vi "Get Cursor X positions.vi"(8 "error in":errorcluster, 11 "XY Graph Ref":refnum<vi>) -> (0 "error out":errorcluster, 1 "Cursors":cluster{"Left":dbl, "Right":dbl, "Span":dbl}, 2 "Right":dbl, 3 "Left":dbl)   [LabVIEW 2015, in "Teaching View.lvlib" / "Teaching View XControl.xctl"]
doc: "Gets the x positions of the right and left cursors of the timeline graph"
uses:
  Teaching View XControl.xctl
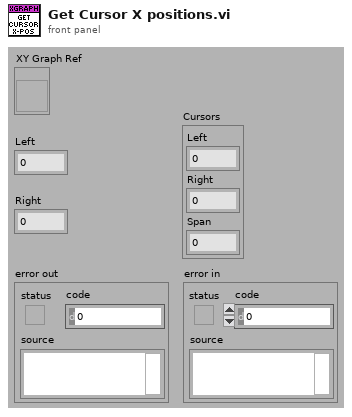
[diagram p1: front panel]
types:
  T1 = cluster{"left":i16, "top":i16, "right":i16, "bottom":i16}
  T2 = cluster{"Cursor.Cursor X":dbl, "Cursor.Cursor X":dbl, dbl}
  T3 = cluster{"Cursor.Cursor X":dbl, "Cursor.Cursor X":dbl}
  T4 = cluster{"XScale.Maximum":dbl, "XScale.Maximum":dbl}
  T5 = cluster{"XScale.Minimum":dbl, "XScale.Minimum":dbl}
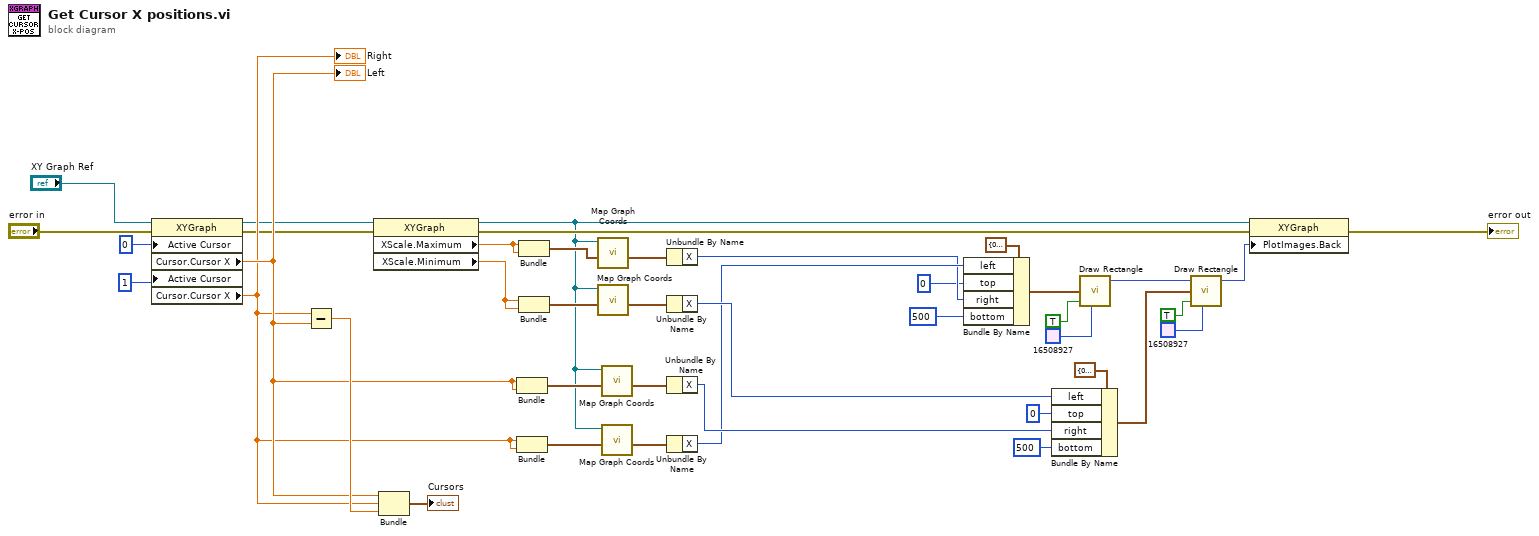
[diagram p0: block diagram]
diagram:
  n1 = property class="XYGraph"(reference="XY Graph Ref", error in="error in", "Active Cursor"=u32 0, "Active Cursor"=u32 1) -> (reference out=w1:refnum<vi>, error out=w2:errorcluster, "Cursor.Cursor X"=w18:dbl, "Cursor.Cursor X"=w17:dbl)
  "Left" <- w18
  "Right" <- w17
  n2 = Subtract(x=w17, y=w18) -> (x-y=w33:dbl)
  n3 = property on="Property Node" class="XYGraph"(reference=w1, error in=w2) -> (reference out=w19:refnum<vi>, error out=w35:errorcluster, "XScale.Maximum"=w39:dbl, "XScale.Minimum"=w38:dbl)
  n4 = Bundle("Cursor.Cursor X"=w18, "Cursor.Cursor X"=w17, w33) -> (→"Cursors":T2)  [unwired: 1 in]
  n5 = Bundle("Cursor.Cursor X"=w18, "Cursor.Cursor X"=w18) -> (w27:T3)  [unwired: 1 in]
  n6 = Bundle("Cursor.Cursor X"=w17, "Cursor.Cursor X"=w17) -> (w26:T3)  [unwired: 1 in]
  n7 = Bundle("XScale.Maximum"=w39, "XScale.Maximum"=w39) -> (w22:T4)  [unwired: 1 in]
  n8 = Bundle("XScale.Minimum"=w38, "XScale.Minimum"=w38) -> (w30:T5)  [unwired: 1 in]
  n9 = call "Map Graph Coords.vi"("XY"=w22, "XY Graph Ref"=w19) -> ("Coords"=w23:cluster{"X":i32, "Y":i32})  [unwired: 8 in, 1 out]
  n10 = call "Map Graph Coords.vi"("XY"=w30, "XY Graph Ref"=w19) -> ("Coords"=w31:cluster{"X":i32, "Y":i32})  [unwired: 8 in, 1 out]
  n11 = call "Map Graph Coords.vi"("XY"=w27, "XY Graph Ref"=w19) -> ("Coords"=w28:cluster{"X":i32, "Y":i32})  [unwired: 8 in, 1 out]
  n12 = call "Map Graph Coords.vi"("XY"=w26, "XY Graph Ref"=w19) -> ("Coords"=w25:cluster{"X":i32, "Y":i32})  [unwired: 8 in, 1 out]
  n13 = Unbundle By Name(w23) -> ("X"=w21:i32)
  n14 = Unbundle By Name(w31) -> ("X"=w32:i32)
  n15 = Unbundle By Name(w28) -> ("X"=w29:i32)
  n16 = Unbundle By Name(w25) -> ("X"=w24:i32)
  n17 = Bundle By Name(cluster=T1 {"left"=0, "top"=0, "right"=0, "bottom"=0} ("rect"), "left"=w24, "top"=i16 0 ("left"), "right"=w21, "bottom"=i16 500) -> (w16:T1)
  n18 = Bundle By Name(cluster=T1 {"left"=0, "top"=0, "right"=0, "bottom"=0} ("rect"), "left"=w32, "top"=i16 0 ("left"), "right"=w29, "bottom"=i16 500) -> (w8:T1)
  n19 = call <vilib>:"Draw Rectangle.vi"("rect"=w16, "fill?(F)"=TRUE, "color(black)"=u32 16508927) -> ("new picture"=w10:picture)  [unwired: 6 in]
  n20 = call <vilib>:"Draw Rectangle.vi"("picture"=w10, "rect"=w8, "fill?(F)"=TRUE, "color(black)"=u32 16508927) -> ("new picture"=w9:picture)  [unwired: 5 in]
  n21 = property on="Property Node" class="XYGraph"(reference=w19, error in=w35, "PlotImages.Back"=w9) -> (error out=→"error out":errorcluster)  [unwired: 1 out]
